vi "Switch_Keysight_34934A_SoftFP.vi"(0 "reference in":refnum<class "Switch_Keysight_34934A.lvclass">, 2 "Floating":bool, 5 "error in (no error)":errorcluster) -> (14 "reference out":refnum<class "Switch_Keysight_34934A.lvclass">, 19 "error out":errorcluster)   [LabVIEW 2022 SP3, in "Switch_Keysight_34934A.lvlib" / "Switch_Keysight_34934A.lvclass"]
uses:
  Switch_Keysight_34934A.lvclass
  <vilib>/picture/picture.llb/imagedata.ctl
  Components/ViPER.lvlibp/ViPER.lvclass
  C:/Projects/Medulla/ViPER/Examples/Flux_Capacitor_Tester/Components/ViPER.lvlibp/ViPER.lvclass
panel:
  in  "Tree":string(tree)
  in  "Disconnect":bool
  in  "M2L":bool[][](array[boolean])
  in  "M2H":bool[][](array[boolean])
  in  "M1L":bool[][](array[boolean])
  in  "M1H":bool[][](array[boolean])
  in  "Connect":bool
  in  "Disconnect":bool
  out "String":string
  # "M1H"
  # "M2H"
  # "M1L"
  # "M2L"
  # "1"
  # "2"
  # "3"
  # "4"
  # "1"
  # "2"
  # "3"
  # "4"
  # "1"
  # "2"
  # "3"
  # "4"
  # "1"
  # "2"
  # "3"
  # "4"
  # "1"
  # "2"
  # "3"
  # "4"
  # "1"
  # "2"
  # "3"
  # "4"
  # "1"
  # "2"
  # "3"
  # "4"
  # "1"
  # "2"
  # "3"
  # "4"
  # "1"
  # "2"
  # "3"
  # "4"
  # "5"
  # "6"
  # "7"
  # "8"
  # "9"
  # "10"
  # "11"
  # "12"
  # "13"
  # "14"
  # "15"
  # "16"
  # "17"
  # "18"
  # "19"
  # "20"
  # "21"
  # "22"
  # "23"
  # "24"
  # "25"
  # "26"
  # "27"
  # "28"
  # "29"
  # "30"
  # "31"
  # "32"
  # "1"
  # "2"
  # "3"
  # "4"
  # "5"
  # "6"
  # "7"
  # "8"
  # "9"
  # "10"
  # "11"
  # "12"
  # "13"
  # "14"
  # "15"
  # "16"
  # "17"
  # "18"
  # "19"
  # "20"
  # "21"
  # "22"
  # "23"
  # "24"
  # "25"
  # "26"
  # "27"
  # "28"
  # "29"
  # "30"
  # "31"
  # "32"
  # "1"
  # "2"
  # "3"
  # "4"
  # "5"
  # "6"
  # "7"
  # "8"
  # "9"
  # "10"
  # "11"
  # "12"
  # "13"
  # "14"
  # "15"
  # "16"
  # "17"
  # "18"
  # "19"
  # "20"
  # "21"
  # "22"
  # "23"
  # "24"
  # "25"
  # "26"
  # "27"
  # "28"
  # "29"
  # "30"
  # "31"
  # "32"
  # "1"
  # "2"
  # "3"
  # "4"
  # "5"
  # "6"
  # "7"
  # "8"
  # "9"
  # "10"
  # "11"
  # "12"
  # "13"
  # "14"
  # "15"
  # "16"
  # "17"
  # "18"
  # "19"
  # "20"
  # "21"
  # "22"
  # "23"
  # "24"
  # "25"
  # "26"
  # "27"
  # "28"
  # "29"
  # "30"
  # "31"
  # "32"
  # "1"
  # "2"
  # "3"
  # "4"
  # "5"
  # "6"
  # "7"
  # "8"
  # "9"
  # "10"
  # "11"
  # "12"
  # "13"
  # "14"
  # "15"
  # "16"
  # "17"
  # "18"
  # "19"
  # "20"
  # "21"
  # "22"
  # "23"
  # "24"
  # "25"
  # "26"
  # "27"
  # "28"
  # "29"
  # "30"
  # "31"
  # "32"
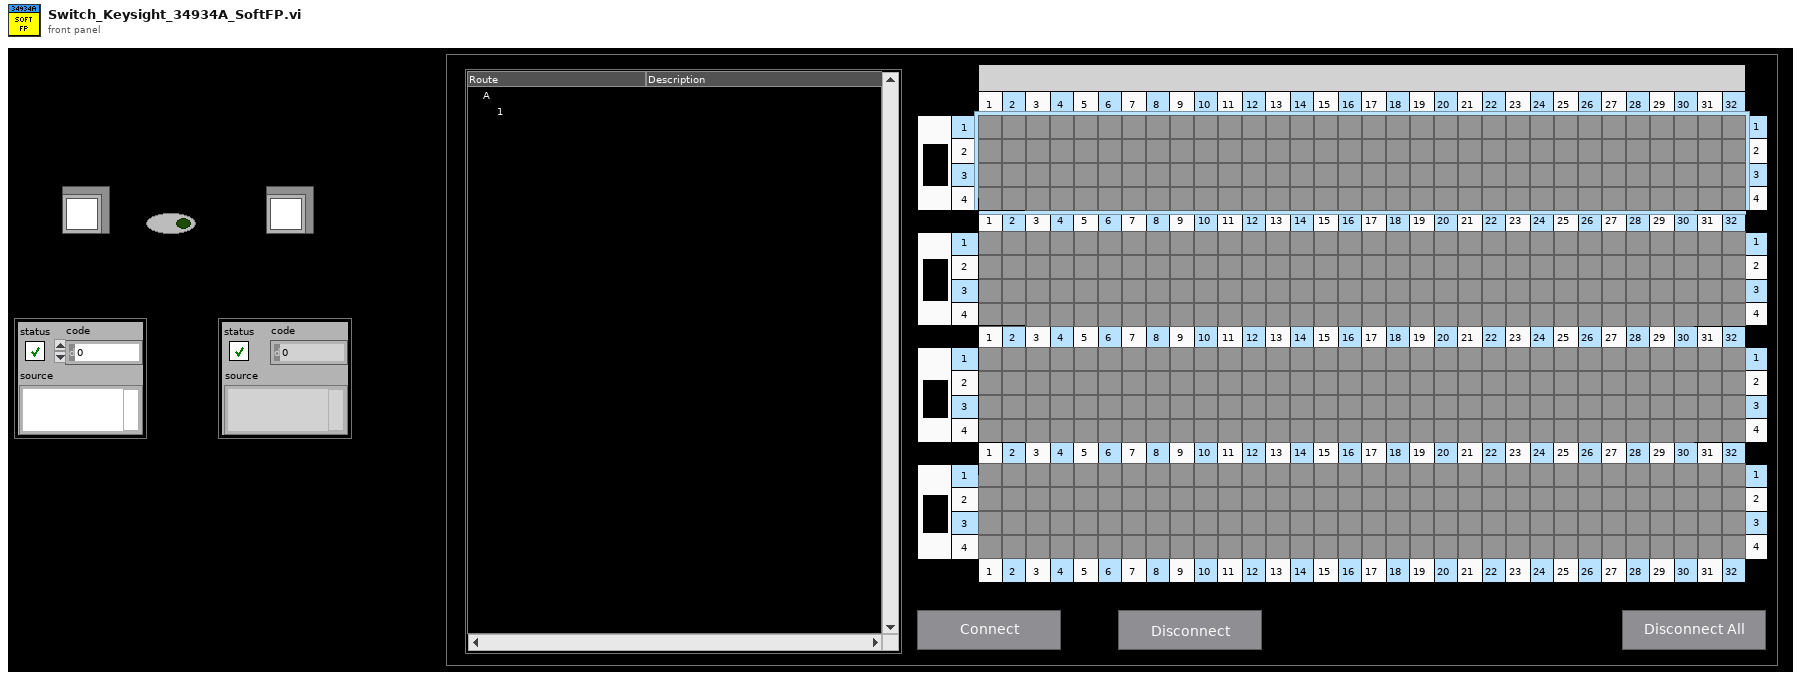
[diagram p1: front panel]
types:
  T1 = enum32{"Invalid", "Standard", "Closed", "Hidden", "Minimized", "Maximized"}
  T2 = typedef "imagedata.ctl" = cluster{"image type":i32, "image depth":i32, "image":u8[], "mask":u8[], "colors":u32[], "Rectangle":cluster{"left":i16, "top":i16, "right":i16, "bottom":i16}}
  T3 = typedef "Switch_Keysight_34934A.lvlib/Switch_Keysight_34934A.lvclass/ObjectAttributes.ctl" = cluster{"Config":T4, "VISA ref":refnum<visa-resource-name>, "M1H":bool[][], "M2H":bool[][], "M1L":bool[][], "M2L":bool[][], "route":string, "State":bool[], "StateModBit":bool[], "UpdateEvent":refnum<user-event>}
  T4 = typedef "Switch_Keysight_34934A.lvlib/Switch_Keysight_34934A.lvclass/Config.ctl" = cluster{"VISA":refnum<visa-resource-name>, "Slot":i32, "SwitchMap":cluster{"Name":string, "Route":string[], "UnRoute":string[], "Description":string, "Group":string, "IsGroup":bool}[], "Sim":bool}
  T5 = cluster{"Name":string, "Route":string[], "UnRoute":string[], "Description":string, "Group":string, "IsGroup":bool}[]
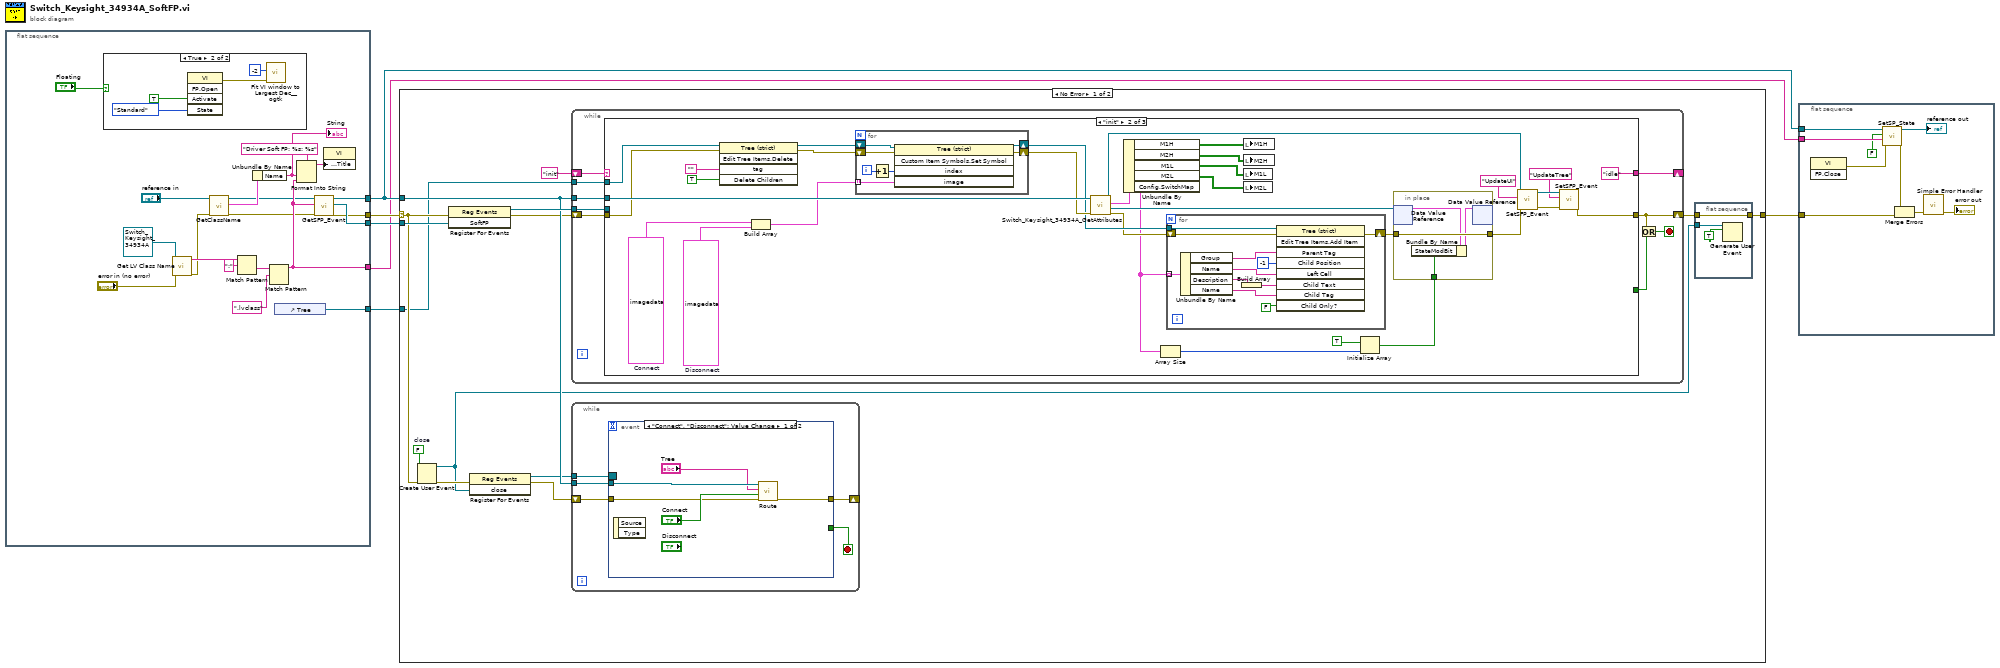
[diagram p0: block diagram]
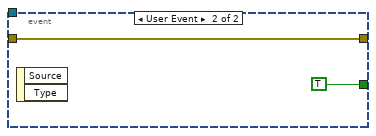
[diagram p3: hidden frame]
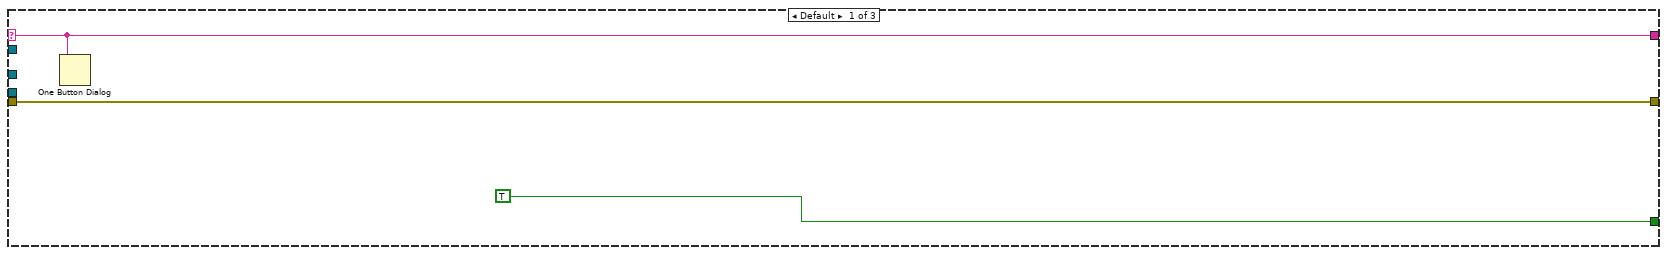
[diagram p4: hidden frame]
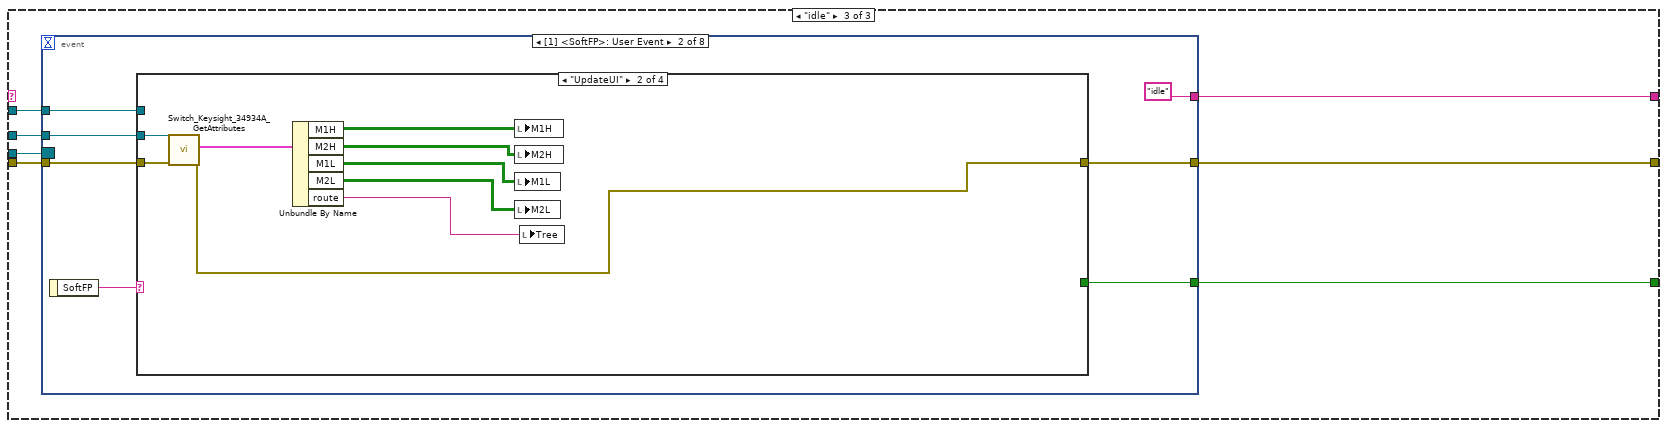
[diagram p5: hidden frame]
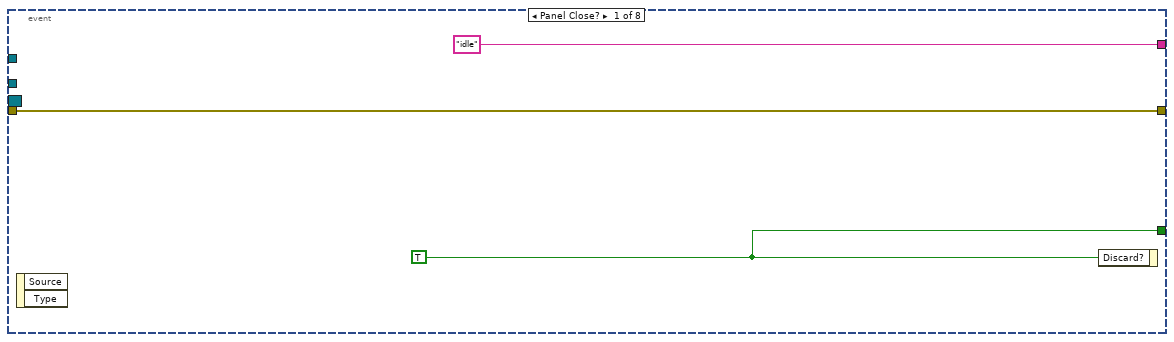
[diagram p6: hidden frame]
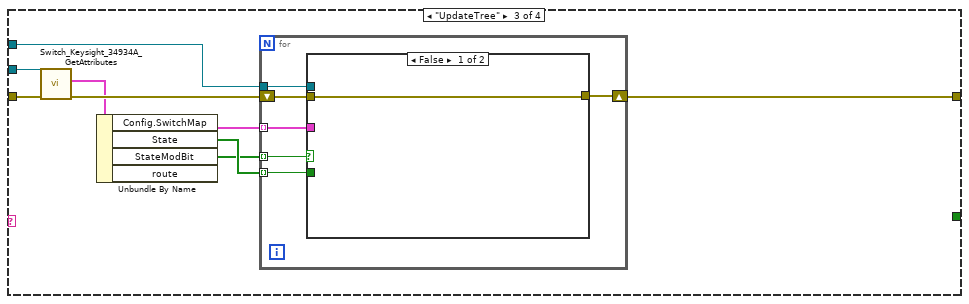
[diagram p8: hidden frame]
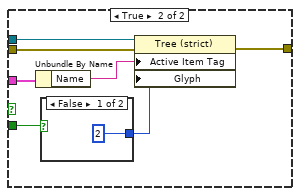
[diagram p9: hidden frame]
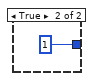
[diagram p10: hidden frame]
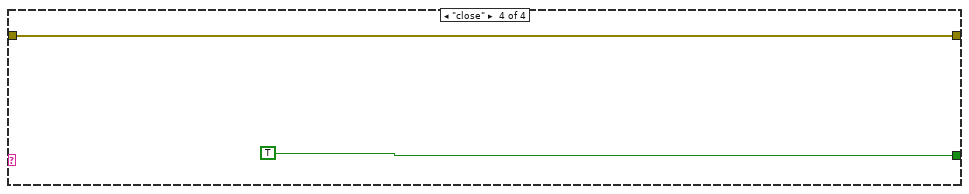
[diagram p11: hidden frame]
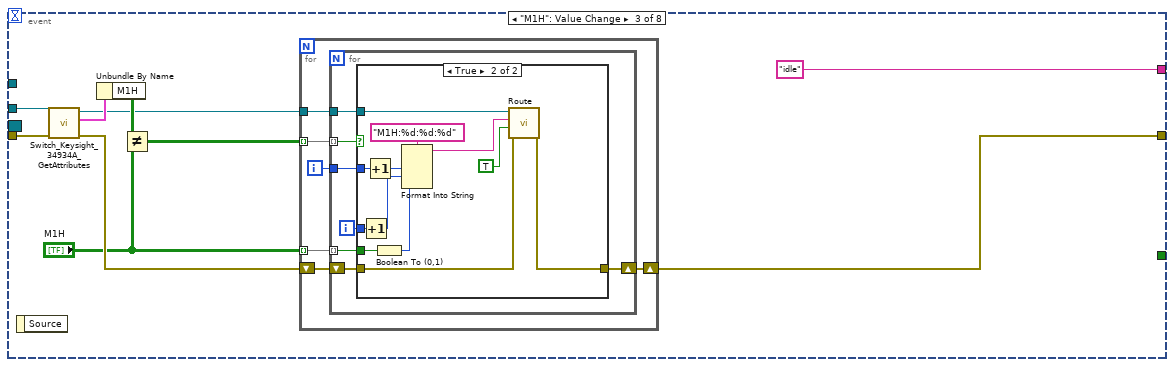
[diagram p12: hidden frame]
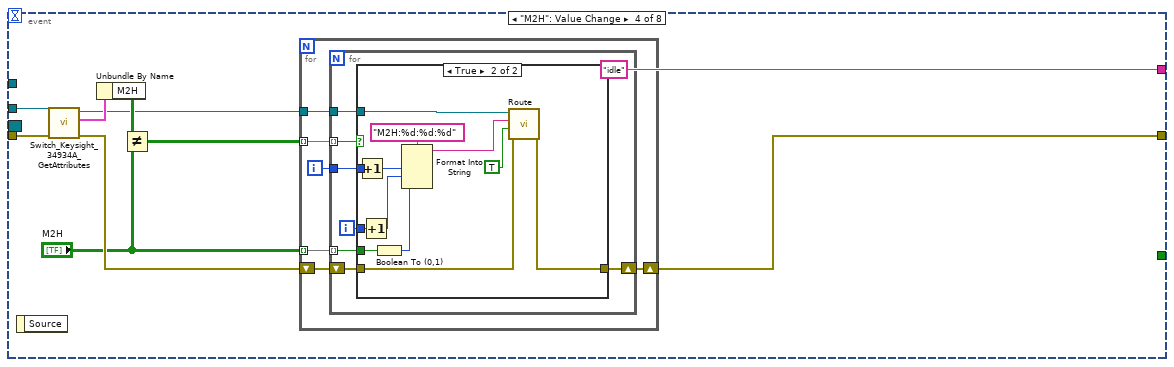
[diagram p14: hidden frame]
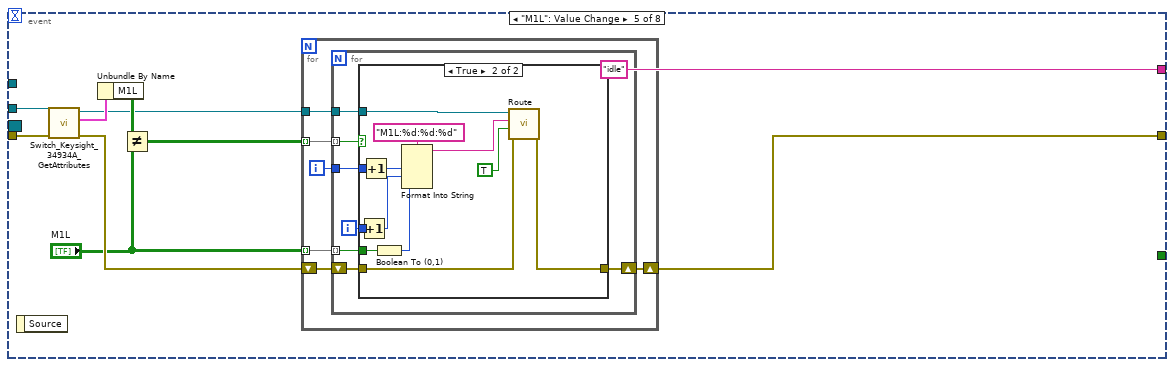
[diagram p16: hidden frame]
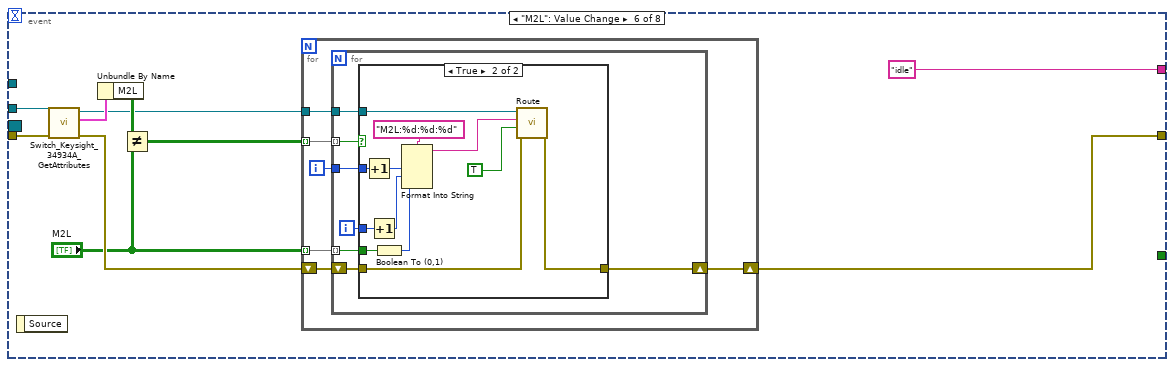
[diagram p18: hidden frame]
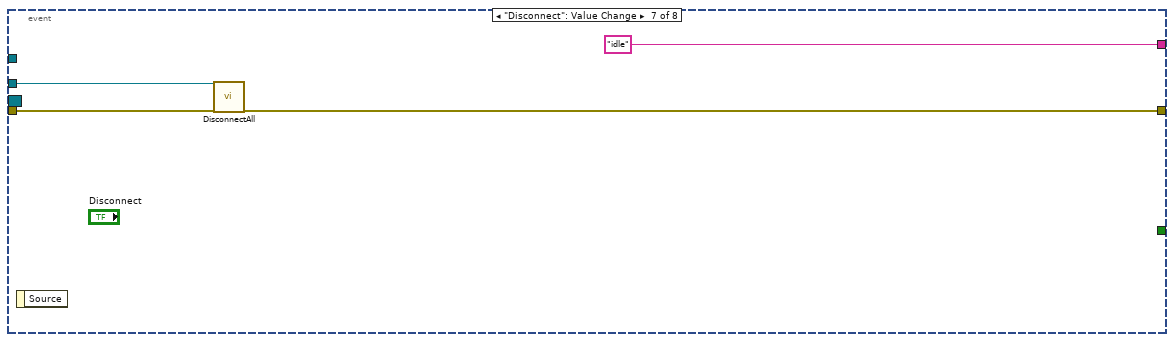
[diagram p20: hidden frame]
diagram:
  n1 = flat-sequence {
    tunnel: [w23] -> w6
    tunnel: [w22] -> w3
    tunnel: [w26] -> w4
    tunnel: [w15] -> w2
    tunnel: [w7] -> w1
    frame #0 {
      n2 = case shown="True" "Floating" {
        frame False {
        }
        frame True {
          n3 = invoke class="VI" method="FP.Open"("Activate"=TRUE ("Activate?"), "State"=T1."Standard") -> (error out=w27:errorcluster)  [unwired: 3 in, 4 out]
          n4 = call <userlib>:"Fit VI window to Largest Dec__ogtk.vi"("error in (no error)"=w27, "border spacing (2 px)"=-2) -> ()  [unwired: 4 in, 2 out]
        }
      }
      n5 = call <vilib>:"Get LV Class Name.vi"("error in (no error)"="error in (no error)", "object"=refnum<class "Switch_Keysight_34934A.lvclass"> refnum ("reference")) -> ("error out"=w14:errorcluster, "class name"=w20:string)  [unwired: 8 in]
      n6 = call "GetClassName.vi"("error in (no error)"=w14, "reference in"="reference in") -> ("error out"=w13:errorcluster, "Details"=w12:cluster{"Name":string, "Class":string}, "reference out"=w10:refnum<class "Switch_Keysight_34934A.lvclass">)  [unwired: 7 in]
      n7 = Match Pattern(string=w20, regular expression=":") -> (after substring=w18:string)  [unwired: 1 in, 3 out]
      n8 = Unbundle By Name(w12) -> ("Name"=w8:string)
      "String" <- w8
      n9 = Match Pattern(string=w18, regular expression=".lvclass") -> (before substring=w15:string)  [unwired: 1 in, 3 out]
      n10 = control-ref of="Tree"() -> (w7:refnum<vi>)
      n11 = Format Into String(format string="Driver Soft FP: %s: %s", w8, w15) -> (resulting string=w25:string)  [unwired: 2 in, 1 out]
      n12 = call-dynamic "GetSFP_Event.vi"("error in (no error)"=w13, "Ancestor"=w15, "reference in"=w10) -> ("error out"=w23:errorcluster, "SoftFP"=w26:refnum<user-event>, "reference out"=w22:refnum<class "Switch_Keysight_34934A.lvclass">)  [unwired: 6 in]
      n13 = property class="VI"("Front Panel.Title"=w25) -> ()  [unwired: 2 in, 2 out]
    }
  }
  n14 = case shown="No Error" w6 {
    selector: w6 -> [w36 w330]
    tunnel: [w33 w330] -> w5
    tunnel: w3 -> [w41 _]
    tunnel: w4 -> [w44 _]
    tunnel: w1 -> [w31 _]
    frame No Error {
      w37 = FALSE  # close
      n15 = Create User Event(user event datatype=w37, error in=w36) -> (user event=w32:refnum<user-event>, error out=w35:errorcluster)
      n16 = register-events(error in=w36, w44) -> (reference out=w43:refnum<event-registration>, error out=w39:errorcluster)  [unwired: 1 in]
      n17 = register-events(error in=w35, w32) -> (reference out=w40:refnum<event-registration>, error out=w38:errorcluster)  [unwired: 1 in]
      n18 = while {
        shift-right: [w51] -> _
        shift-left: w38 -> [w52]
        tunnel: w41 -> [w50]
        tunnel: w40 -> [w49]
        stop <- w48 stop-if-true
        n19 = event shown="[0] \"Connect\", \"Disconnect\": Value Change" {
          selector: w49 -> [_ _]
          dyn-events: _ -> [_ _]
          timeout: _ -> [_ _]
          tunnel: w52 -> [w54 w59]
          tunnel: [w57 w59] -> w51
          tunnel: w50 -> [w56 _]
          tunnel: [_ TRUE] -> w48
          event "Connect", "Disconnect": Value Change {
            n20 = event-data() -> ()  [unwired: 1 in, 2 out]
            n21 = call-dynamic "Route.vi"("error in (no error)"=w54, "Connect"="Connect", "channel 1"="Tree", "reference in"=w56) -> ("error out"=w57:errorcluster)  [unwired: 6 in, 1 out]
          }
          event User Event {
            n22 = event-data() -> ()  [unwired: 1 in, 2 out]
          }
        }
      }
      n23 = while {
        shift-right: [w65] -> w34
        shift-left: w39 -> [w68]
        tunnel: w43 -> [w67]
        tunnel: w41 -> [w66]
        shift-right: [w61] -> _
        shift-left: "init" -> [w62]
        tunnel: w31 -> [w60]
        stop <- w64 stop-if-true
        n24 = case shown="\"init\"" w62 {
          selector: w62 -> [w69 _ _]
          tunnel: w68 -> [w70 w87 w132]
          tunnel: w67 -> [_ _ w131]
          tunnel: w66 -> [_ w102 w130]
          tunnel: [w70 w81 w129] -> w65
          tunnel: [TRUE ("Discard?") _ w128] -> w63
          tunnel: [w69 "idle" w127] -> w61
          tunnel: w60 -> [_ w86 w126]
          frame Default {
            n25 = One Button Dialog(message=w69) -> ()  [unwired: 1 in, 1 out]
          }
          frame "init" {
            w83 = T2 {"image type"=0, "image depth"=32, "image"=[255, 0, 0, 0, 255, 0, 0, 0, 255, 0, 0, 0, 255, 0, 0, 0, 255, 0, 0, 0, 255, 0, 0, 0, 255, 0, 0, 0, 255, 0, 0, 0, 255, 0, 0, 0, 255, 0, 0, 0, 255, 0, 0, 0, 255, 0, 0, 0, 255, 0, 0, 0, 255, 0, 0, 0, 255, 0, 0, 0, 255, 0, 0, 0, 255, 0, 0, 0, 255, 0, 0, 0, 255, 0, 0, 0, 255, 0, 0, 0, 255, 136, 118, 121, 255, 113, 64, 72, 255, 122, 43, 52, 255, 138, 48, 56, 255, 136, 46, 54, 255, 120, 40, 49, 255, 113, 64, 72, 255, 0, 0, 0, 255, 0, 0, 0, 255, 0, 0, 0, 255, 0, 0, 0, 255, 0, 0, 0, 255, 0, 0, 0, 255, 0, 0, 0, 255, 0, 0, 0, 255, 119, 79, 86, 255, 137, 51, 59, 255, 189, 85, 89, 255, 201, 100, 103, 255, 201, 102, 105, 255, 198, 94, 97, 255, 194, 81, 84, 255, 180, 64, 69, 255, 130, 39, 48, 255, 121, 84, 90, 255, 0, 0, 0, 255, 0, 0, 0, 255, 0, 0, 0, 255, 0, 0, 0, 255, 0, 0, 0, 255, 119, 79, 86, 255, 161, 64, 71, 255, 202, 103, 106, 255, 209, 123, 126, 255, 211, 129, 132, 255, 208, 122, 125, 255, 203, 105, 109, 255, 196, 87, 90, 255, 192, 74, 78, 255, 189, 68, 72, 255, 150, 47, 54, 255, 121, 86, 92, 255, 0, 0, 0, 255, 0, 0, 0, 255, 0, 0, 0, 255, 136, 118, 121, 255, 137, 51, 59, 255, 202, 103, 106, 255, 211, 129, 132, 255, 214, 140, 142, 255, 212, 133, 136, 255, 205, 113, 116, 255, 196, 88, 92, 255, 190, 68, 72, 255, 188, 63, 67, 255, 189, 68, 72, 255, 190, 69, 73, 255, 129, 40, 49, 255, 0, 0, 0, 255, 0, 0, 0, 255, 0, 0, 0, 255, 113, 64, 72, 255, 188, 84, 88, 255, 207, 120, 122, 255, 213, 135, 138, 255, 211, 131, 133, 255, 205, 112, 115, 255, 195, 85, 88, 255, 186, 59, 63, 255, 181, 44, 48, 255, 181, 45, 49, 255, 187, 61, 65, 255, 191, 73, 77, 255, 177, 62, 67, 255, 114, 68, 76, 255, 0, 0, 0, 255, 0, 0, 0, 255, 122, 42, 51, 255, 199, 94, 98, 255, 207, 118, 121, 255, 207, 119, 122, 255, 201, 102, 105, 255, 193, 78, 82, 255, 185, 54, 58, 255, 178, 36, 41, 255, 176, 28, 33, 255, 178, 34, 39, 255, 185, 55, 59, 255, 192, 74, 78, 255, 191, 71, 75, 255, 117, 40, 50, 255, 0, 0, 0, 255, 0, 0, 0, 255, 136, 44, 53, 255, 197, 89, 92, 255, 201, 100, 103, 255, 197, 88, 92, 255, 189, 67, 71, 255, 182, 47, 52, 255, 177, 33, 38, 255, 174, 25, 30, 255, 174, 23, 28, 255, 177, 32, 37, 255, 185, 54, 58, 255, 192, 75, 79, 255, 192, 75, 79, 255, 128, 36, 46, 255, 0, 0, 0, 255, 0, 0, 0, 255, 134, 40, 49, 255, 192, 75, 79, 255, 192, 77, 80, 255, 187, 60, 64, 255, 180, 41, 46, 255, 176, 29, 34, 255, 174, 24, 28, 255, 174, 22, 27, 255, 174, 25, 30, 255, 179, 37, 42, 255, 187, 61, 65, 255, 194, 81, 85, 255, 193, 78, 81, 255, 128, 37, 46, 255, 0, 0, 0, 255, 0, 0, 0, 255, 119, 35, 45, 255, 188, 63, 67, 255, 187, 61, 66, 255, 182, 46, 51, 255, 177, 32, 36, 255, 174, 25, 30, 255, 174, 24, 29, 255, 175, 27, 32, 255, 178, 36, 40, 255, 184, 53, 57, 255, 192, 76, 80, 255, 197, 90, 93, 255, 193, 79, 82, 255, 117, 42, 52, 255, 0, 0, 0, 255, 0, 0, 0, 255, 112, 63, 71, 255, 176, 52, 57, 255, 186, 59, 63, 255, 183, 50, 54, 255, 180, 40, 44, 255, 178, 36, 40, 255, 179, 38, 42, 255, 182, 46, 50, 255, 187, 60, 64, 255, 193, 79, 83, 255, 199, 96, 99, 255, 199, 96, 99, 255, 178, 70, 75, 255, 115, 72, 79, 255, 0, 0, 0, 255, 0, 0, 0, 255, 0, 0, 0, 255, 129, 34, 44, 255, 186, 59, 63, 255, 187, 61, 66, 255, 186, 59, 63, 255, 186, 59, 63, 255, 188, 64, 68, 255, 192, 75, 78, 255, 197, 89, 92, 255, 201, 102, 105, 255, 202, 104, 107, 255, 197, 89, 93, 255, 127, 44, 53, 255, 0, 0, 0, 255, 0, 0, 0, 255, 0, 0, 0, 255, 0, 0, 0, 255, 121, 84, 90, 255, 149, 44, 51, 255, 188, 65, 69, 255, 191, 72, 76, 255, 193, 78, 82, 255, 195, 85, 89, 255, 198, 93, 97, 255, 201, 100, 104, 255, 201, 101, 104, 255, 197, 90, 93, 255, 148, 54, 62, 255, 124, 93, 98, 255, 0, 0, 0, 255, 0, 0, 0, 255, 0, 0, 0, 255, 0, 0, 0, 255, 0, 0, 0, 255, 121, 85, 91, 255, 128, 38, 47, 255, 177, 61, 66, 255, 191, 73, 77, 255, 193, 79, 83, 255, 195, 83, 86, 255, 194, 82, 86, 255, 178, 71, 76, 255, 127, 44, 53, 255, 124, 93, 98, 255, 0, 0, 0, 255, 0, 0, 0, 255, 0, 0, 0, 255, 0, 0, 0, 255, 0, 0, 0, 255, 0, 0, 0, 255, 0, 0, 0, 255, 0, 0, 0, 255, 114, 68, 76, 255, 117, 40, 49, 255, 129, 37, 46, 255, 128, 37, 46, 255, 117, 42, 52, 255, 115, 72, 79, 255, 0, 0, 0, 255, 0, 0, 0, 255, 0, 0, 0, 255, 0, 0, 0, 255, 0, 0, 0, 255, 0, 0, 0, 255, 0, 0, 0, 255, 0, 0, 0, 255, 0, 0, 0, 255, 0, 0, 0, 255, 0, 0, 0, 255, 0, 0, 0, 255, 0, 0, 0, 255, 0, 0, 0, 255, 0, 0, 0, 255, 0, 0, 0, 255, 0, 0, 0, 255, 0, 0, 0, 255, 0, 0, 0, 255, 0, 0, 0, 255, 0, 0, 0], "mask"=[255, 255, 255, 255, 255, 255, 255, 255, 255, 255, 255, 255, 255, 255, 255, 255, 255, 255, 255, 255, 255, 255, 255, 255, 255, 255, 255, 255, 255, 255, 255, 255], "colors"=[], "Rectangle"={"left"=0, "top"=0, "right"=16, "bottom"=16}}  # Disconnect
            w84 = T2 {"image type"=0, "image depth"=32, "image"=array[1024 elements], "mask"=[255, 255, 255, 255, 255, 255, 255, 255, 255, 255, 255, 255, 255, 255, 255, 255, 255, 255, 255, 255, 255, 255, 255, 255, 255, 255, 255, 255, 255, 255, 255, 255], "colors"=[], "Rectangle"={"left"=0, "top"=0, "right"=16, "bottom"=16}}  # Connect
            n26 = invoke class="Tree (strict)" method="Edit Tree Items.Delete"(reference=w86, error in=w87, "tag"="", "Delete Children"=TRUE ("Delete Children?")) -> (reference out=w85:refnum<vi>, error out=w88:errorcluster)  [unwired: 1 in, 3 out]
            n27 = Build Array(w84, w83) -> (w94:T2[])
            n28 = for {
              tunnel: w94 -> [w122] mode=indexing
              shift-right: [w121] -> w93
              shift-left: w88 -> [w124]
              shift-right: [w119] -> w92
              shift-left: w85 -> [w120]
              i -> [w125]
              n29 = Increment(x=w125) -> (x+1=w123:i32)
              n30 = invoke class="Tree (strict)" method="Custom Item Symbols.Set Symbol"(reference=w120, error in=w124, "index"=w123, "image"=w122) -> (reference out=w119:refnum<vi>, error out=w121:errorcluster)  [unwired: 1 in, 3 out]
            }
            n31 = call "Switch_Keysight_34934A_GetAttributes.vi"("error in (no error)"=w93, "reference in"=w102) -> ("error out"=w91:errorcluster, "DataRef"=w76:refnum<data-value>, "Data"=w101:T3, "reference out"=w95:refnum<class "Switch_Keysight_34934A.lvclass">)  [unwired: 6 in]
            n32 = Unbundle By Name(w101) -> ("M1H"=w100:bool[][], "M2H"=w99:bool[][], "M1L"=w98:bool[][], "M2L"=w97:bool[][], "Config.SwitchMap"=w75:T5)
            n33 = Array Size(array=w75) -> (size(s)=w74:i32)
            n34 = for {
              tunnel: w75 -> [w118] mode=indexing
              tunnel: w92 -> [w111]
              shift-right: [w109] -> w78
              shift-left: w91 -> [w110]
              n35 = Unbundle By Name(w118) -> ("Group"=w117:string, "Name"=w113:string, "Description"=w115:string, "Name"=w108:string)
              n36 = Build Array(w115) -> (w114:string[])
              n37 = invoke class="Tree (strict)" method="Edit Tree Items.Add Item"(reference=w111, error in=w110, "Parent Tag"=w117, "Child Position"=-1, "Left Cell"=w113, "Child Text"=w114, "Child Tag"=w108, "Child Only?"=FALSE) -> (error out=w109:errorcluster)  [unwired: 1 in, 8 out]
            }
            n38 = local write "M1H"(w100) -> ()
            n39 = local write "M2H"(w99) -> ()
            n40 = local write "M1L"(w98) -> ()
            n41 = local write "M2L"(w97) -> ()
            n42 = Initialize Array(TRUE, w74) -> (w72:bool[])
            n43 = in-place {
              in-place-border: w78 -> [w107]
              in-place-border: [w107] -> w77
              in-place-border: w72 -> [w104]
              n44 = in-place-dvr #1(w76) -> (w106:T3)  [unwired: 1 out]
              n45 = Bundle By Name(cluster=w106, "StateModBit"=w104) -> (w105:T3)
              n46 = in-place-dvr #1(w105) -> ()  [unwired: 2 out]
            }
            n47 = call-dynamic "SetSFP_Event.vi"("error in (no error)"=w77, "msg"="UpdateUI", "reference in"=w95) -> ("error out"=w82:errorcluster, "reference out"=w80:refnum<class "Switch_Keysight_34934A.lvclass">)  [unwired: 7 in]
            n48 = call-dynamic "SetSFP_Event.vi"("error in (no error)"=w82, "msg"="UpdateTree", "reference in"=w80) -> ("error out"=w81:errorcluster)  [unwired: 7 in, 1 out]
          }
          frame "idle" {
            n49 = event shown="[1] <SoftFP>: User Event" {
              selector: w131 -> [_ _ _ _ _ _ _ _]
              dyn-events: _ -> [_ _ _ _ _ _ _ _]
              timeout: _ -> [_ _ _ _ _ _ _ _]
              tunnel: w132 -> [w135 w142 w188 w224 w260 w296 w327 w329]
              tunnel: [w135 w140 w181 w217 w253 w289 w325 w329] -> w129
              tunnel: [w134 w139 _ _ _ _ _ _] -> w128
              tunnel: w130 -> [_ w137 w187 w223 w259 w295 w326 _]
              tunnel: ["idle" "idle" "idle" "idle" "idle" "idle" "idle" "idle"] -> w127
              tunnel: w126 -> [_ w136 _ _ _ _ _ _]
              event Panel Close? {
                w134 = TRUE ("Discard?")
                n50 = event-data() -> ()  [unwired: 1 in, 2 out]
                n51 = event-data("Discard?"=w134) -> ()  [unwired: 1 in, 1 out]
              }
              event User Event {
                n52 = event-data() -> ("SoftFP"=w141:string)  [unwired: 1 in]
                n53 = case shown="\"UpdateUI\"" w141 {
                  tunnel: w142 -> [w143 w151 w159 w179]
                  tunnel: [w143 w145 w153 w179] -> w140
                  tunnel: [_ _ _ TRUE ("Discard?")] -> w139
                  tunnel: w137 -> [_ w152 w158 _]
                  tunnel: w136 -> [_ _ w161 _]
                  frame Default {
                  }
                  frame "UpdateUI" {
                    n54 = call "Switch_Keysight_34934A_GetAttributes.vi"("error in (no error)"=w151, "reference in"=w152) -> ("error out"=w145:errorcluster, "Data"=w150:T3)  [unwired: 6 in, 2 out]
                    n55 = Unbundle By Name(w150) -> ("M1H"=w149:bool[][], "M2H"=w148:bool[][], "M1L"=w147:bool[][], "M2L"=w146:bool[][], "route"=w144:string)
                    n56 = local write "M1H"(w149) -> ()
                    n57 = local write "M2H"(w148) -> ()
                    n58 = local write "M1L"(w147) -> ()
                    n59 = local write "M2L"(w146) -> ()
                    n60 = local write "Tree"(w144) -> ()
                  }
                  frame "UpdateTree" {
                    n61 = call "Switch_Keysight_34934A_GetAttributes.vi"("error in (no error)"=w159, "reference in"=w158) -> ("error out"=w160:errorcluster, "Data"=w157:T3)  [unwired: 6 in, 2 out]
                    n62 = Unbundle By Name(w157) -> ("Config.SwitchMap"=w156:T5, "State"=w155:bool[], "StateModBit"=w154:bool[])  [unwired: 1 out]
                    n63 = for {
                      tunnel: w161 -> [w167]
                      tunnel: w156 -> [w166] mode=indexing
                      tunnel: w155 -> [w165] mode=indexing
                      shift-right: [w163] -> w153
                      shift-left: w160 -> [w164]
                      tunnel: w154 -> [w162] mode=indexing
                      n64 = case shown="False" w162 {
                        tunnel: w167 -> [_ w175]
                        tunnel: w166 -> [_ w174]
                        tunnel: w165 -> [_ w172]
                        tunnel: w164 -> [w168 w170]
                        tunnel: [w168 w169] -> w163
                        frame False {
                        }
                        frame True {
                          n65 = Unbundle By Name(w174) -> ("Name"=w173:string)
                          n66 = case shown="False" w172 {
                            tunnel: [2 1] -> w171
                            frame False {
                            }
                            frame True {
                            }
                          }
                          n67 = property class="Tree (strict)"(reference=w175, error in=w170, "Active Item Tag"=w173, "Glyph"=w171) -> (error out=w169:errorcluster)  [unwired: 1 out]
                        }
                      }
                    }
                  }
                  frame "close" {
                  }
                }
              }
              event "M1H": Value Change {
                n68 = event-data() -> ()  [unwired: 1 in, 1 out]
                n69 = call "Switch_Keysight_34934A_GetAttributes.vi"("error in (no error)"=w188, "reference in"=w187) -> ("error out"=w183:errorcluster, "Data"=w186:T3, "reference out"=w182:refnum<class "Switch_Keysight_34934A.lvclass">)  [unwired: 6 in, 1 out]
                n70 = Unbundle By Name(w186) -> ("M1H"=w185:bool[][])
                n71 = Not Equal?(x=w185, y="M1H") -> (x != y?=w184:bool[][])
                n72 = for {
                  tunnel: w184 -> [w195] mode=indexing
                  tunnel: "M1H" -> [w193] mode=indexing
                  shift-right: [w191] -> w181
                  shift-left: w183 -> [w194]
                  tunnel: w182 -> [w192]
                  i -> [w190]
                  n73 = for {
                    tunnel: w195 -> [w202] mode=indexing
                    tunnel: w193 -> [w200] mode=indexing
                    tunnel: w192 -> [w199]
                    shift-right: [w198] -> w191
                    shift-left: w194 -> [w201]
                    tunnel: w190 -> [w197]
                    i -> [w196]
                    n74 = case shown="True" w202 {
                      tunnel: w201 -> [w203 w215]
                      tunnel: w200 -> [_ w209]
                      tunnel: w199 -> [_ w210]
                      tunnel: [w203 w214] -> w198
                      tunnel: w197 -> [_ w213]
                      tunnel: w196 -> [_ w211]
                      frame False {
                      }
                      frame True {
                        n75 = Increment(x=w211) -> (x+1=w205:i32)
                        n76 = Increment(x=w213) -> (x+1=w206:i32)
                        n77 = Boolean To (0,1)(Boolean=w209) -> (0, 1=w208:i16)
                        n78 = Format Into String(format string="M1H:%d:%d:%d", w206, w205, w208) -> (resulting string=w207:string)  [unwired: 2 in, 1 out]
                        n79 = call-dynamic "Route.vi"("error in (no error)"=w215, "Connect"=TRUE, "channel 1"=w207, "reference in"=w210) -> ("error out"=w214:errorcluster)  [unwired: 6 in, 1 out]
                      }
                    }
                  }
                }
              }
              event "M2H": Value Change {
                n80 = event-data() -> ()  [unwired: 1 in, 1 out]
                n81 = call "Switch_Keysight_34934A_GetAttributes.vi"("error in (no error)"=w224, "reference in"=w223) -> ("error out"=w219:errorcluster, "Data"=w222:T3, "reference out"=w218:refnum<class "Switch_Keysight_34934A.lvclass">)  [unwired: 6 in, 1 out]
                n82 = Unbundle By Name(w222) -> ("M2H"=w221:bool[][])
                n83 = Not Equal?(x=w221, y="M2H") -> (x != y?=w220:bool[][])
                n84 = for {
                  tunnel: w220 -> [w231] mode=indexing
                  tunnel: "M2H" -> [w229] mode=indexing
                  shift-right: [w227] -> w217
                  shift-left: w219 -> [w230]
                  tunnel: w218 -> [w228]
                  i -> [w226]
                  n85 = for {
                    tunnel: w231 -> [w238] mode=indexing
                    tunnel: w229 -> [w236] mode=indexing
                    tunnel: w228 -> [w235]
                    shift-right: [w234] -> w227
                    shift-left: w230 -> [w237]
                    tunnel: w226 -> [w233]
                    i -> [w232]
                    n86 = case shown="True" w238 {
                      tunnel: w237 -> [w239 w251]
                      tunnel: w236 -> [_ w245]
                      tunnel: w235 -> [_ w246]
                      tunnel: [w239 w250] -> w234
                      tunnel: w233 -> [_ w249]
                      tunnel: w232 -> [_ w247]
                      frame False {
                      }
                      frame True {
                        n87 = Increment(x=w249) -> (x+1=w242:i32)
                        n88 = Increment(x=w247) -> (x+1=w241:i32)
                        n89 = Boolean To (0,1)(Boolean=w245) -> (0, 1=w244:i16)
                        n90 = Format Into String(format string="M2H:%d:%d:%d", w242, w241, w244) -> (resulting string=w243:string)  [unwired: 2 in, 1 out]
                        n91 = call-dynamic "Route.vi"("error in (no error)"=w251, "Connect"=TRUE, "channel 1"=w243, "reference in"=w246) -> ("error out"=w250:errorcluster)  [unwired: 6 in, 1 out]
                      }
                    }
                  }
                }
              }
              event "M1L": Value Change {
                n92 = event-data() -> ()  [unwired: 1 in, 1 out]
                n93 = call "Switch_Keysight_34934A_GetAttributes.vi"("error in (no error)"=w260, "reference in"=w259) -> ("error out"=w255:errorcluster, "Data"=w258:T3, "reference out"=w254:refnum<class "Switch_Keysight_34934A.lvclass">)  [unwired: 6 in, 1 out]
                n94 = Unbundle By Name(w258) -> ("M1L"=w257:bool[][])
                n95 = Not Equal?(x=w257, y="M1L") -> (x != y?=w256:bool[][])
                n96 = for {
                  tunnel: w256 -> [w267] mode=indexing
                  tunnel: "M1L" -> [w265] mode=indexing
                  shift-right: [w263] -> w253
                  shift-left: w255 -> [w266]
                  tunnel: w254 -> [w264]
                  i -> [w262]
                  n97 = for {
                    tunnel: w267 -> [w274] mode=indexing
                    tunnel: w265 -> [w272] mode=indexing
                    tunnel: w264 -> [w271]
                    shift-right: [w270] -> w263
                    shift-left: w266 -> [w273]
                    tunnel: w262 -> [w269]
                    i -> [w268]
                    n98 = case shown="True" w274 {
                      tunnel: w273 -> [w275 w287]
                      tunnel: w272 -> [_ w281]
                      tunnel: w271 -> [_ w282]
                      tunnel: [w275 w286] -> w270
                      tunnel: w269 -> [_ w285]
                      tunnel: w268 -> [_ w283]
                      frame False {
                      }
                      frame True {
                        n99 = Increment(x=w283) -> (x+1=w277:i32)
                        n100 = Increment(x=w285) -> (x+1=w278:i32)
                        n101 = Boolean To (0,1)(Boolean=w281) -> (0, 1=w280:i16)
                        n102 = Format Into String(format string="M1L:%d:%d:%d", w278, w277, w280) -> (resulting string=w279:string)  [unwired: 2 in, 1 out]
                        n103 = call-dynamic "Route.vi"("error in (no error)"=w287, "Connect"=TRUE, "channel 1"=w279, "reference in"=w282) -> ("error out"=w286:errorcluster)  [unwired: 6 in, 1 out]
                      }
                    }
                  }
                }
              }
              event "M2L": Value Change {
                n104 = event-data() -> ()  [unwired: 1 in, 1 out]
                n105 = call "Switch_Keysight_34934A_GetAttributes.vi"("error in (no error)"=w296, "reference in"=w295) -> ("error out"=w291:errorcluster, "Data"=w294:T3, "reference out"=w290:refnum<class "Switch_Keysight_34934A.lvclass">)  [unwired: 6 in, 1 out]
                n106 = Unbundle By Name(w294) -> ("M2L"=w293:bool[][])
                n107 = Not Equal?(x=w293, y="M2L") -> (x != y?=w292:bool[][])
                n108 = for {
                  tunnel: w292 -> [w303] mode=indexing
                  tunnel: "M2L" -> [w301] mode=indexing
                  shift-right: [w299] -> w289
                  shift-left: w291 -> [w302]
                  tunnel: w290 -> [w300]
                  i -> [w298]
                  n109 = for {
                    tunnel: w303 -> [w310] mode=indexing
                    tunnel: w301 -> [w308] mode=indexing
                    tunnel: w300 -> [w307]
                    shift-right: [w306] -> w299
                    shift-left: w302 -> [w309]
                    tunnel: w298 -> [w305]
                    i -> [w304]
                    n110 = case shown="True" w310 {
                      tunnel: w309 -> [w311 w323]
                      tunnel: w308 -> [_ w317]
                      tunnel: w307 -> [_ w318]
                      tunnel: [w311 w322] -> w306
                      tunnel: w305 -> [_ w321]
                      tunnel: w304 -> [_ w319]
                      frame False {
                      }
                      frame True {
                        n111 = Increment(x=w321) -> (x+1=w314:i32)
                        n112 = Increment(x=w319) -> (x+1=w313:i32)
                        n113 = Boolean To (0,1)(Boolean=w317) -> (0, 1=w316:i16)
                        n114 = Format Into String(format string="M2L:%d:%d:%d", w314, w313, w316) -> (resulting string=w315:string)  [unwired: 2 in, 1 out]
                        n115 = call-dynamic "Route.vi"("error in (no error)"=w323, "Connect"=TRUE, "channel 1"=w315, "reference in"=w318) -> ("error out"=w322:errorcluster)  [unwired: 6 in, 1 out]
                      }
                    }
                  }
                }
              }
              event "Disconnect": Value Change {
                n116 = event-data() -> ()  [unwired: 1 in, 1 out]
                n117 = call-dynamic "DisconnectAll.vi"("reference in"=w326, "error in (no error)"=w327) -> ("error out"=w325:errorcluster)  [unwired: 16 in, 1 out]
              }
              event Timeout {
                n118 = event-data() -> ()  [unwired: 1 in, 2 out]
              }
            }
          }
        }
        n119 = Or(x=w65, y=w63) -> (x .or. y?=w64:bool)
      }
      n120 = flat-sequence {
        tunnel: w34 -> [w47]
        tunnel: [w47] -> w33
        tunnel: w32 -> [w46]
        frame #0 {
          n121 = Generate User Event(user event=w46, event data cluster=TRUE) -> ()  [unwired: 2 in, 2 out]
        }
      }
    }
    frame Error {
    }
  }
  n122 = flat-sequence {
    tunnel: w5 -> [w337]
    tunnel: w3 -> [w332]
    tunnel: w2 -> [w334]
    frame #0 {
      n123 = invoke class="VI" method="FP.Close"() -> (error out=w336:errorcluster)  [unwired: 3 in, 2 out]
      n124 = call "SetSP_State.vi"("error in (no error)"=w336, "Ancestor"=w334, "SP Open"=FALSE, "reference in"=w332) -> ("error out"=w335:errorcluster, "reference out"=→"reference out":refnum<class "Switch_Keysight_34934A.lvclass">)  [unwired: 6 in]
      n125 = Merge Errors(w335, w337) -> (w339:errorcluster)
      n126 = call <vilib>:"Simple Error Handler.vi"("error in (no error)"=w339) -> ("error out"=→"error out":errorcluster)  [unwired: 4 in, 4 out]
    }
  }
